vi "LED_Set2.vi"(10 "board PF L":bool[](array[boolean])) -> ()   [LabVIEW 2018]
uses:
  Subvi/Global.vi
panel:
  out "数组 2":string[](array[string])
  out "数组":bool[](array[boolean])
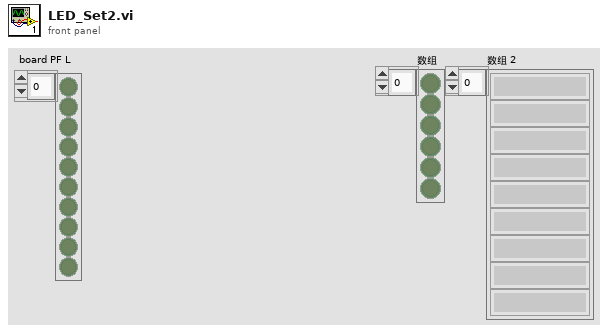
[diagram p1: front panel]
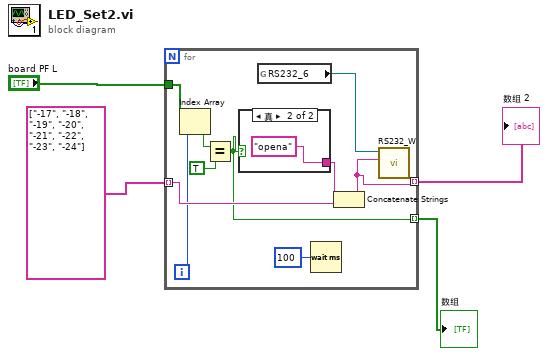
[diagram p0: block diagram]
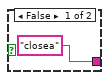
[diagram p2: hidden frame]
diagram:
  n1 = for {
    tunnel: "board PF L" -> [w11]
    tunnel: string[] ["-17", "-18", "-19", "-20", "-21", "-22", "-23", "-24"] -> [w12] mode=indexing
    tunnel: [w7] -> w2 mode=indexing
    tunnel: [w6] -> w1 mode=indexing
    i -> [w10]
    n2 = Index Array(array=w11, index=w10) -> (element=w8:bool)
    n3 = Equal?(x=w8, y=TRUE) -> (x = y?=w7:bool)
    n4 = case shown="真" w7 {
      tunnel: ["closea" ("字符串") "opena" ("字符串")] -> w13
      frame False {
      }
      frame True {
      }
    }
    n5 = global read "Global.vi" "RS232_6"() -> (w14:refnum<visa-resource-name>)
    n6 = Wait (ms)(milliseconds to wait=u32 100 ("等待时间（毫秒）")) -> ()  [unwired: 1 out]
    n7 = Concatenate Strings(w13, w12) -> (w6:string)
    n8 = call "RS232_W.vi"("CMD"=w6, "VISA资源名称"=w14) -> ()  [unwired: 7 in, 3 out]
  }
  "数组" <- w2
  "数组 2" <- w1
